vi "IsSameItem.vi"(8 "error in (no error)":errorcluster, 9 "Compare to item":refnum<class "ILabVIEWItem.lvclass">, 11 "CLabVIEWItem in":refnum<class "CLabVIEWItem.lvclass">) -> (0 "error out":errorcluster, 2 "Is same?":bool, 3 "CLabVIEWItem out":refnum<class "CLabVIEWItem.lvclass">)   [LabVIEW 2020, in "LabVIEWItem.lvlib" / "CLabVIEWItem.lvclass"]
uses:
  CLabVIEWItem.lvclass
  obj/Addons/LabVIEWObjectInterfaces.lvlibp/LabVIEWObjectInterfaces/ILabVIEWItem/ILabVIEWItem.lvclass
  CLabVIEWItem.lvclass/CLabVIEWItem.ctl
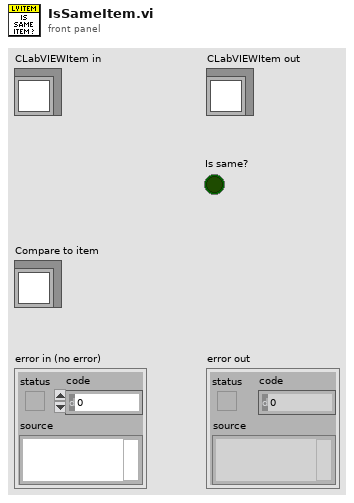
[diagram p1: front panel]
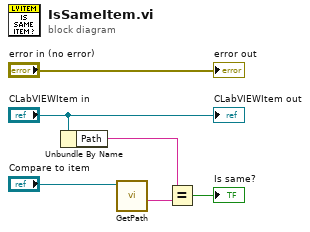
[diagram p0: block diagram]
diagram:
  n1 = Unbundle By Name("CLabVIEWItem in") -> ("Path"=w2:string)
  n2 = call-dynamic "GetPath.vi"("ILabVIEWItem in"="Compare to item") -> ("Path"=w3:string)  [unwired: 8 in, 2 out]
  n3 = Equal?(x=w2, y=w3) -> (x = y?=→"Is same?":bool)
  "error out" <- "error in (no error)"
  "CLabVIEWItem out" <- "CLabVIEWItem in"
